vi "Unibot - State Machine Controller.vi"(3 "dt (s)":dbl=-1.0 format="%.3f", 4 "Limit":dbl=10.0, 5 "Up Optimal Gain":dbl[](array[numeric])=[-16.4615, -16.2422, -3.1287, -2.0658], 6 "Mode":T1(ring), 7 "Setpoint":dbl(knob) scale=-1.0..1.0, 8 "Enable":bool, 9 "Kill":bool, 10 "PID gains":T2={"proportional gain (Kc)"=1.0, "integral time (Ti, min)"=0.01, "derivative time (Td, min)"=0.0} {"derivative time (Td, min)" format="%.3f"; "integral time (Ti, min)" format="%.3f"; "proportional gain (Kc)" format="%.3f"}, 11 "States":dbl[](array[numeric])=[-0.0012566370614359172, -0.8117875416876026, 0.0, 0.0]) -> (0 "Status":string="Kill", 2 "Control Effort":dbl(knob) scale=-1000.0..1000.0)   [LabVIEW 2012]
uses:
  Unibot - States.ctl
  <vilib>/addons/Control Design/_Implementation/CD State Feedback Controller (Single Output).vi
  <vilib>/addons/control/pid/pid.llb/PID (DBL).vi
  <vilib>/addons/Control Design/_Implementation/NI_CD_Implementation.lvlib
  <vilib>/addons/control/pid/NI_PID_pid.lvlib
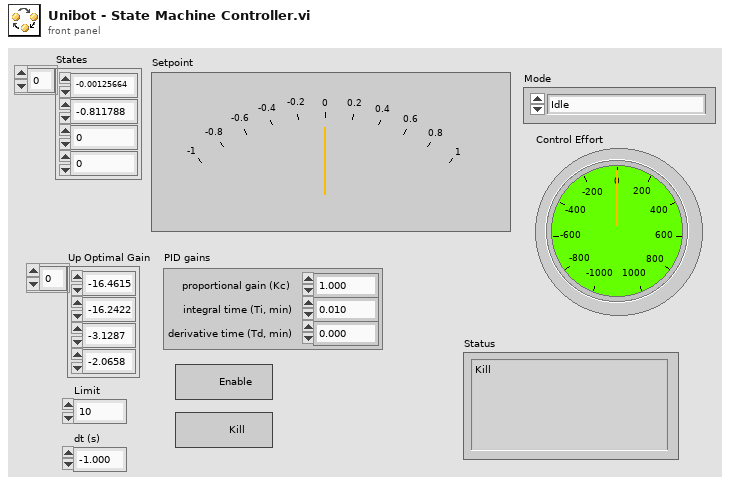
[diagram p1: front panel]
types:
  T1 = enum16{"Idle", "Linear Balance", "Proportional Balance", "PID Balance", "Emergency"}
  T2 = cluster{"proportional gain (Kc)":dbl, "integral time (Ti, min)":dbl, "derivative time (Td, min)":dbl}
  T3 = typedef "Unibot - States.ctl" = enum16{"Idle", "Linear Balance", "Proportional Balance", "PID Balance", "Emergency"}
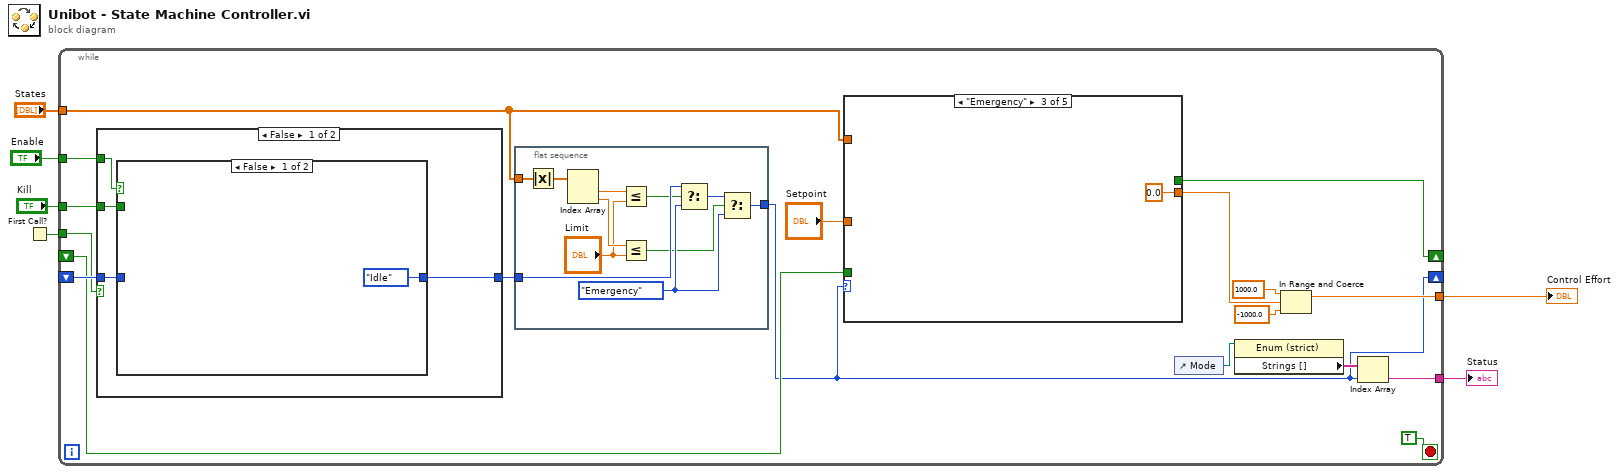
[diagram p0: block diagram]
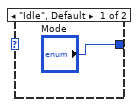
[diagram p3: hidden frame]
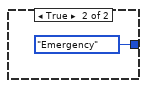
[diagram p4: hidden frame]
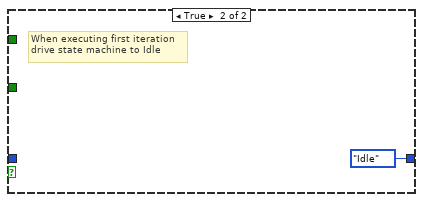
[diagram p5: hidden frame]
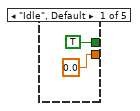
[diagram p6: hidden frame]
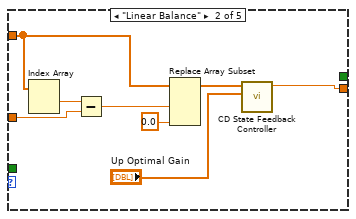
[diagram p7: hidden frame]
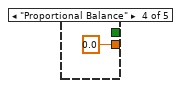
[diagram p8: hidden frame]
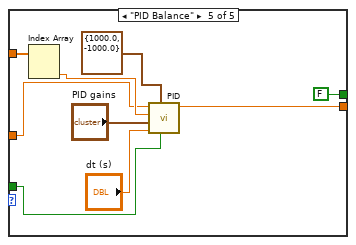
[diagram p9: hidden frame]
diagram:
  n1 = First Call?() -> (First Call?: T/F=w3:bool)
  n2 = while {
    tunnel: "States" -> [w19]
    tunnel: [w16] -> w1
    shift-right: [w7] -> _
    shift-left: _ -> [w22]
    tunnel: [w12] -> w5
    tunnel: "Kill" -> [w23]
    tunnel: w3 -> [w21]
    tunnel: "Enable" -> [w20]
    shift-right: [w10] -> _
    shift-left: _ -> [w11]
    stop <- TRUE stop-if-true
    n3 = case shown="False" w21 {
      tunnel: w23 -> [w39 _]
      tunnel: w22 -> [w38 _]
      tunnel: w20 -> [w37 _]
      tunnel: [w36 Unibot_-_States."Idle" ("Enum")] -> w18
      frame False {
        n4 = case shown="False" w37 {
          tunnel: w39 -> [_ w43]
          tunnel: w38 -> [_ w41]
          tunnel: [Unibot_-_States."Idle" ("Enum") w42] -> w36
          frame False {
          }
          frame True {
            n5 = case shown="False" w43 {
              tunnel: [w44 Unibot_-_States."Emergency" ("Enum")] -> w42
              tunnel: w41 -> [w45 _]
              frame False {
                n6 = case shown="\"Emergency\"" w45 {
                  selector: w45 -> [_ w47]
                  tunnel: ["Mode" w47] -> w44
                  frame "Idle", Default {
                  }
                  frame "Emergency" {
                  }
                }
              }
              frame True {
              }
            }
          }
        }
      }
      frame True {
        # "When executing first iteration\ndrive state machine to Idle"
      }
    }
    n7 = flat-sequence {
      tunnel: w19 -> [w30]
      tunnel: w18 -> [w35]
      tunnel: [w32] -> w7
      frame #0 {
        w33 = Unibot_-_States."Emergency" ("Enum")
        n8 = Absolute Value(x=w30) -> (abs(x)=w31:dbl[])
        n9 = Index Array(array=w31) -> (element #1=w28:dbl, element #2=w29:dbl)  [unwired: 2 in]
        n10 = Less Or Equal?(x=w28, y="Limit") -> (x <= y?=w27:bool)
        n11 = Less Or Equal?(x=w29, y="Limit") -> (x <= y?=w26:bool)
        n12 = Select(t=w35, s=w27, f=w33) -> (s? t:f=w34:T3)
        n13 = Select(t=w34, s=w26, f=w33) -> (s? t:f=w32:T3)
      }
    }
    n14 = case shown="\"Emergency\"" w7 {
      tunnel: w19 -> [_ w56 _ _ w67]
      tunnel: [0.0 w54 0.0 0.0 ("output") w68] -> w17
      tunnel: "Setpoint" -> [_ w53 _ _ w65]
      tunnel: w11 -> [_ _ _ _ w63]
      tunnel: [TRUE ("Enable") _ _ _ FALSE ("Enable")] -> w10
      frame "Idle", Default {
      }
      frame "Linear Balance" {
        n15 = Index Array(array=w56) -> (element #1=w55:dbl)  [unwired: 2 in, 1 out]
        n16 = Subtract(x=w55, y=w53) -> (x-y=w58:dbl)
        n17 = Replace Array Subset(array=w56, new element #1=w58, new element #2=0.0 ("x")) -> (w59:dbl[])  [unwired: 2 in]
        n18 = call-poly <vilib>:"CD State Feedback Controller.vi"("Controller Gain"="Up Optimal Gain", "States"=w59) -> ("Controller Action"=w54:dbl)  [unwired: 1 in, 8 out]
      }
      frame "Emergency" {
      }
      frame "Proportional Balance" {
      }
      frame "PID Balance" {
        n19 = Index Array(array=w67) -> (element #2=w66:dbl)  [unwired: 2 in, 1 out]
        n20 = call-poly <vilib>:"PID.vi"("reinitialize? (F)"=w63, "output range"=cluster{"output high":dbl, "output low":dbl} {"output high"=1000.0, "output low"=-1000.0}, "dt (s)"="dt (s)", "PID gains"="PID gains", "process variable"=w66, "setpoint"=w65) -> ("output"=w68:dbl)  [unwired: 4 in, 1 out]
      }
    }
    n21 = control-ref of="Mode"() -> (w8:refnum<vi>)
    n22 = property class="Enum (strict)"(reference=w8) -> ("Strings []"=w13:string[])  [unwired: 1 in, 2 out]
    n23 = In Range and Coerce(upper limit=1000.0, x=w17, lower limit=-1000.0) -> (coerced(x)=w16:dbl)  [unwired: 1 out]
    n24 = Index Array(array=w13, index=w7) -> (element=w12:string)
  }
  "Control Effort" <- w1
  "Status" <- w5
